vi "Raw Text to 1D String.vi"(8 "Error In":errorcluster, 11 "Relative Path to Input File":string) -> (0 "Error Out":errorcluster, 3 "1D String Array":string[](array[string]))   [LabVIEW 2019]
doc: "Given a relative path, retrieve a 1D string array from an input text file. This assumes Line Feed delimiters."
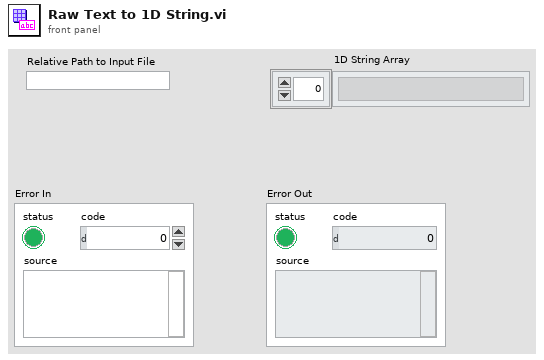
[diagram p1: front panel]
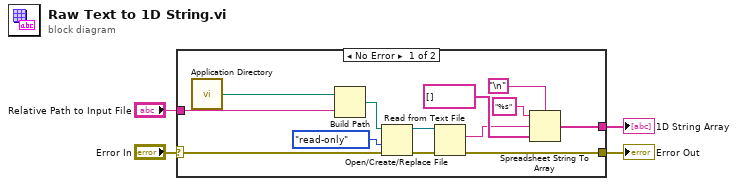
[diagram p0: block diagram]
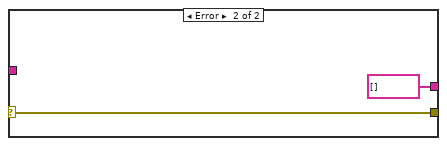
[diagram p2: hidden frame]
diagram:
  n1 = case shown="No Error" "Error In" {
    selector: "Error In" -> [w5 w19]
    tunnel: "Relative Path to Input File" -> [w16 _]
    tunnel: [w8 string[] []] -> w3
    tunnel: [w7 w19] -> w2
    frame No Error {
      n2 = call <vilib>:"Application Directory.vi"() -> ("Application Directory"=w17:path)
      n3 = Build Path(base path=w17, name or relative path=w16) -> (appended path=w15:path)
      n4 = Open/Create/Replace File(file path (use dialog)=w15, error in=w5, access (0:read/write)=enum16{"read/write", "read-only", "write-only"}."read-only") -> (refnum out=w13:refnum<file>, error out=w12:errorcluster)  [unwired: 3 in, 1 out]
      n5 = Read from Text File(file (use dialog)=w13, error in=w12) -> (text=w10:string, error out=w7:errorcluster)  [unwired: 2 in, 2 out]
      n6 = Spreadsheet String To Array(delimiter (Tab)="\n", format string="%s", spreadsheet string=w10, array type (2D Dbl)=string[] []) -> (array=w8:string[])
    }
    frame Error {
    }
  }
  "Error Out" <- w2
  "1D String Array" <- w3
